vi "Global 2.vi"() -> ()   [LabVIEW 2011]
panel:
  out "Test output":T1
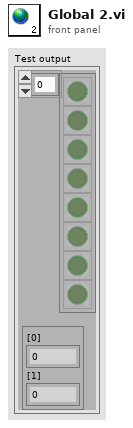
[diagram p1: front panel]
types:
  T1 = cluster{cluster{bool}[], cluster{"[0]":dbl, "[1]":dbl}}
diagram:
